vi "Set RIO Device Settings Dynamic.vi"(0 "Target Info":cluster{"RIO Device":string}={"RIO Device"="rio://192.168.0.2/RIO0"}, 5 "FPGA AutoLoad Mode":T2(radio), 7 "Analog Input Mode":T1(radio), 9 "Synchronize FPGA Clock to PXI_CLK10":bool, 11 "Error In":errorcluster) -> (4 "Target Info Out":cluster{"FPGA Target Resource":string}, 15 "Error Out":errorcluster)   [LabVIEW 2018]
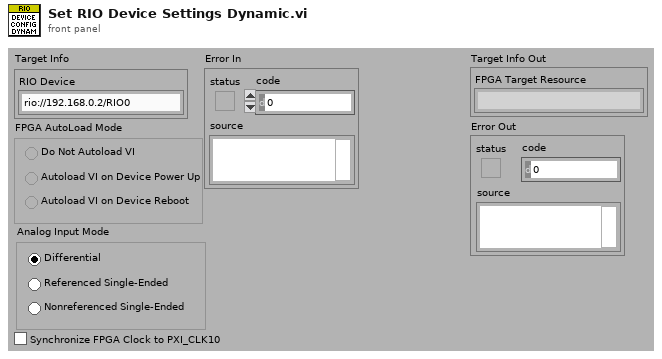
[diagram p1: front panel]
types:
  T1 = enum32{"Differential", "Referenced Single-Ended", "Nonreferenced Single-Ended"}
  T2 = enum32{"Do Not Autoload on Reset", "Autoload on Power-On Reset", "Autoload on Any Device Reset"}
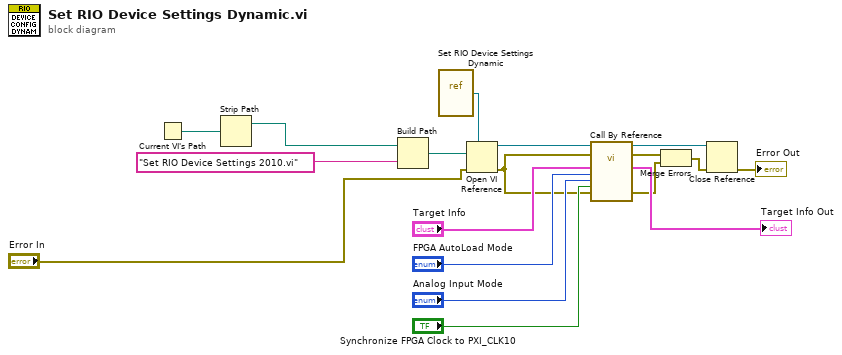
[diagram p0: block diagram]
diagram:
  n1 = Current VI's Path() -> (path=w1:path)
  n2 = Strip Path(path=w1) -> (stripped path=w18:path)  [unwired: 1 out]
  n3 = Build Path(base path=w18, name or relative path="Set RIO Device Settings 2010.vi") -> (appended path=w16:path)
  n4 = vi-ref "Set RIO Device Settings Dynamic.vi"() -> (w15:refnum<vi>)
  n5 = Open VI Reference(type specifier VI Refnum (for type only)=w15, vi path=w16, error in (no error)="Error In") -> (vi reference=w14:refnum<vi>, error out=w2:errorcluster)  [unwired: 3 in]
  n6 = call-by-ref "?"(reference=w14, error in=w2, "Target Info"="Target Info", "FPGA AutoLoad Mode"="FPGA AutoLoad Mode", "Analog Input Mode"="Analog Input Mode", "Synchronize FPGA Clock to PXI_CLK10"="Synchronize FPGA Clock to PXI_CLK10", "Error In"=w2) -> (reference out=w7:refnum<vi>, error out=w6:errorcluster, "Target Info Out"=→"Target Info Out":cluster{"FPGA Target Resource":string}, "Error Out"=w5:errorcluster)  [unwired: 9 in]
  n7 = Merge Errors(w6, w5) -> (w4:errorcluster)
  n8 = Close Reference(reference=w7, error in (no error)=w4) -> (error out=→"Error Out":errorcluster)
